vi "RyanChargeDischargeCycling - Copy.vi"() -> ()   [LabVIEW 2020]
uses:
  <instrlib>/NH Research Regenerative Test Series/Public/Configure/Output Safety.ctl
  <vilib>/DAQmx/read.llb/DAQmx Read (Analog 1D DBL NChan 1Samp).vi
  <vilib>/DAQmx/miscellaneous.llb/DAQmx Fill In Error Info.vi
  <instrlib>/NH Research Regenerative Test Series/Public/Data/Read (Ave Current).vi
  <instrlib>/NH Research Regenerative Test Series/Public/Data/Low Level/Fetch (Ave Voltage).vi
  <instrlib>/NH Research Regenerative Test Series/Public/Data/Low Level/Fetch (Ave True Power).vi
  <instrlib>/NH Research Regenerative Test Series/NH Research Regenerative Test Series.lvlib
panel:
  out "Waveform Chart 2":dbl(graph)
  out "Gauge":dbl(knob) scale=0.0..10.0
  out "Boolean":bool
  out "Waveform Chart":dbl(graph)
  in  "Charge Stop":bool
  in  "Post Discharge Wait Time 2":dbl
  out "Discharge Rest Voltage":dbl
  out "Status Byte Register 4":T1
  out "Post Discharge Wait Time Elaspsed":dbl caption="Elapsed Time (s)"
  in  "Discharge Current":dbl
  out "Cycle Index":dbl
  in  "Cycles":dbl
  in  "Discharge Voltage Setpoint":dbl
  out "Task error out":errorcluster
  out "String":string
  out "Filename Out 3":path caption="Filename Out"
  in  "Discharge Data File Name .lvm":path
  out "Ave Current (A) 3":dbl
  out "Ave Voltage (V) 3":dbl
  out "Ave True Power (W) 3":dbl
  out "Status Byte Register 3":T1
  out "Voltage Compare":dbl
  out "Battemp":dbl
  out "AmbientTemp":dbl
  in  "Post Charge Wait Time":dbl
  out "Charge Rest Voltage":dbl
  out "Status Byte Register 2":T1
  out "WaitElapsed Time (s)":dbl caption="Elapsed Time (s)"
  in  "Output Safety":T2
  out "Filename Out":path
  in  "DAQmx Task Name":refnum<k21>
  in  "Charging Data File Name .lvm":path
  in  "Charge Current Cutoff":dbl
  out "Ave Current (A)":dbl
  out "Ave Voltage (V)":dbl
  out "Ave True Power (W)":dbl
  out "Status Byte Register":T1
  out "Battemp":dbl
  out "AmbientTemp":dbl
  in  "Logical Instrument Number":u32=1
  in  "Charge Current":dbl format="%#.6g"
  in  "Charge Voltage":dbl format="%#.6g"
  in  "Battery Detect Voltage (0V)":dbl format="%#.6g"
  in  "VISA resource name":refnum<visa-resource-name>
  # "T couples need calibration"
  # "Dont know which is which"
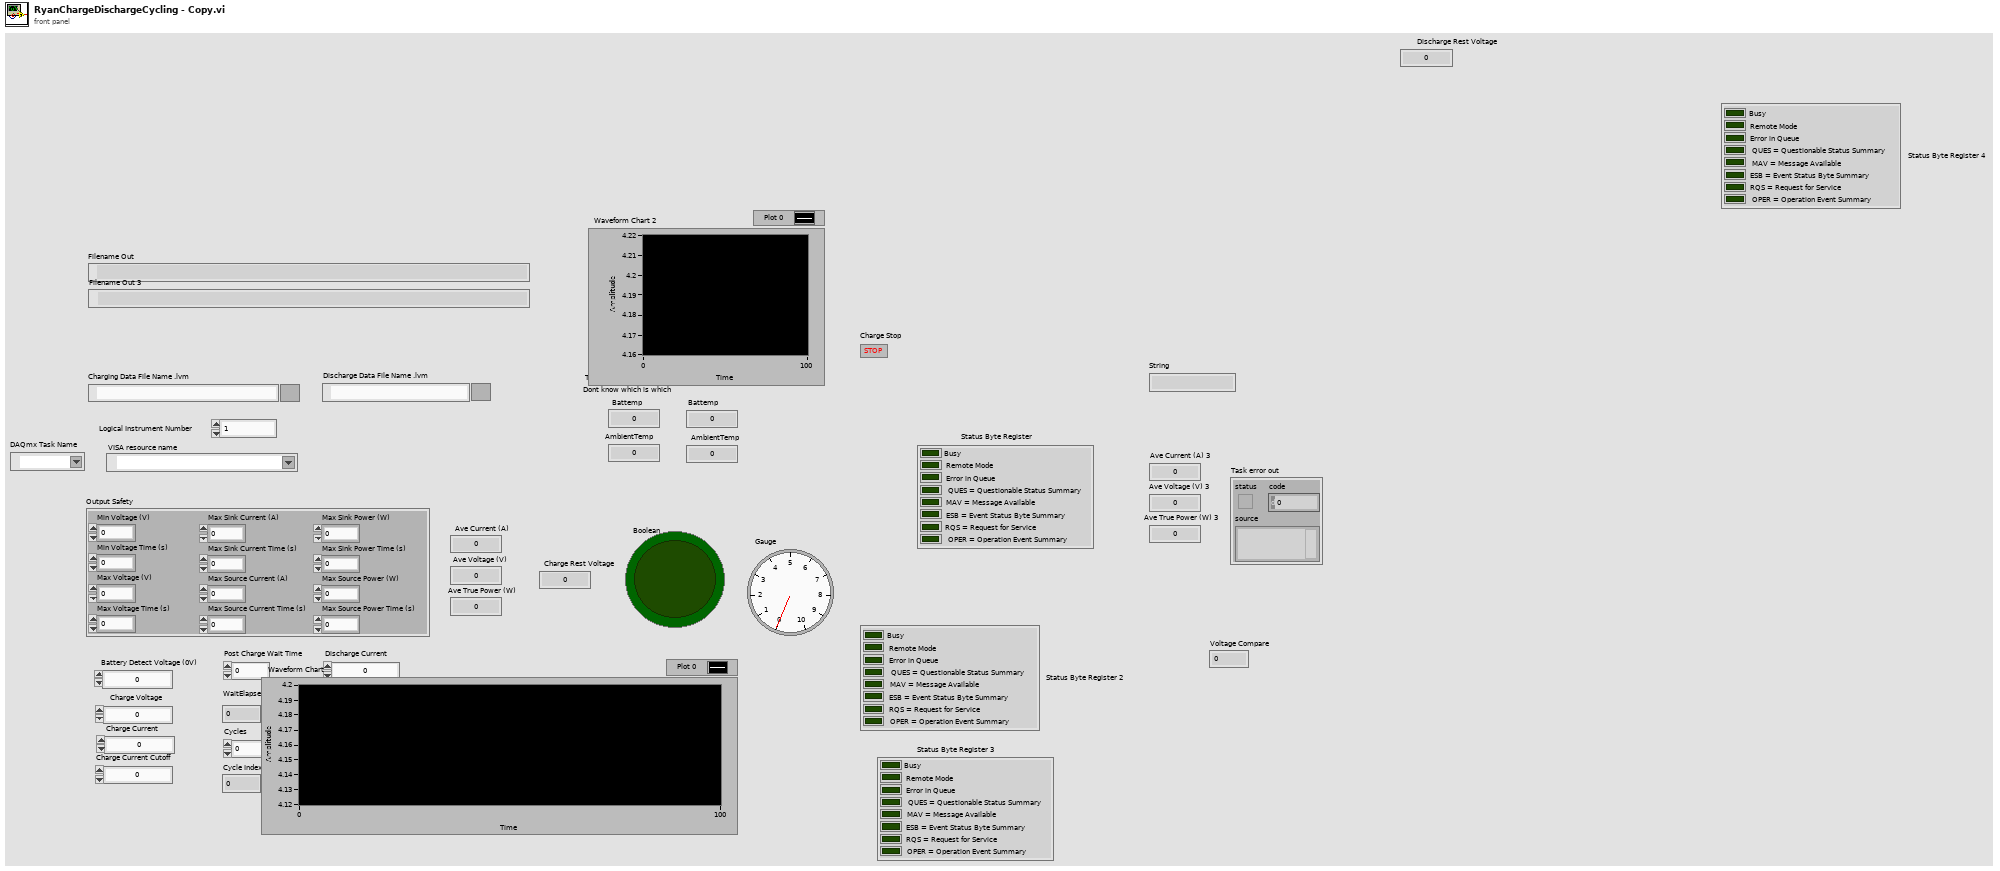
[diagram p1: front panel]
types:
  T1 = cluster{"Busy":bool, "Remote Mode":bool, "Error in Queue":bool, "QUES = Questionable Status Summary":bool, "MAV = Message Available":bool, "ESB = Event Status Byte Summary":bool, "RQS = Request for Service":bool, "OPER = Operation Event Summary":bool}
  T2 = typedef "NH Research Regenerative Test Series.lvlib/Output Safety.ctl" = cluster{"Min Voltage (V)":dbl, "Min Voltage Time (s)":dbl, "Max Voltage (V)":dbl, "Max Voltage Time (s)":dbl, "Max Sink Current (A)":dbl, "Max Sink Current Time (s)":dbl, "Max Source Current (A)":dbl, "Max Source Current Time (s)":dbl, "Max Sink Power (W)":dbl, "Max Sink Power Time (s)":dbl, "Max Source Power (W)":dbl, "Max Source Power Time (s)":dbl}
  T3 = cluster{"data[0]":dbl, "data[1]":dbl, "data[2]":dbl, "data[3]":dbl, "data[4]":dbl, "data[5]":dbl, "data[6]":dbl, "data[7]":dbl, "data[8]":dbl}
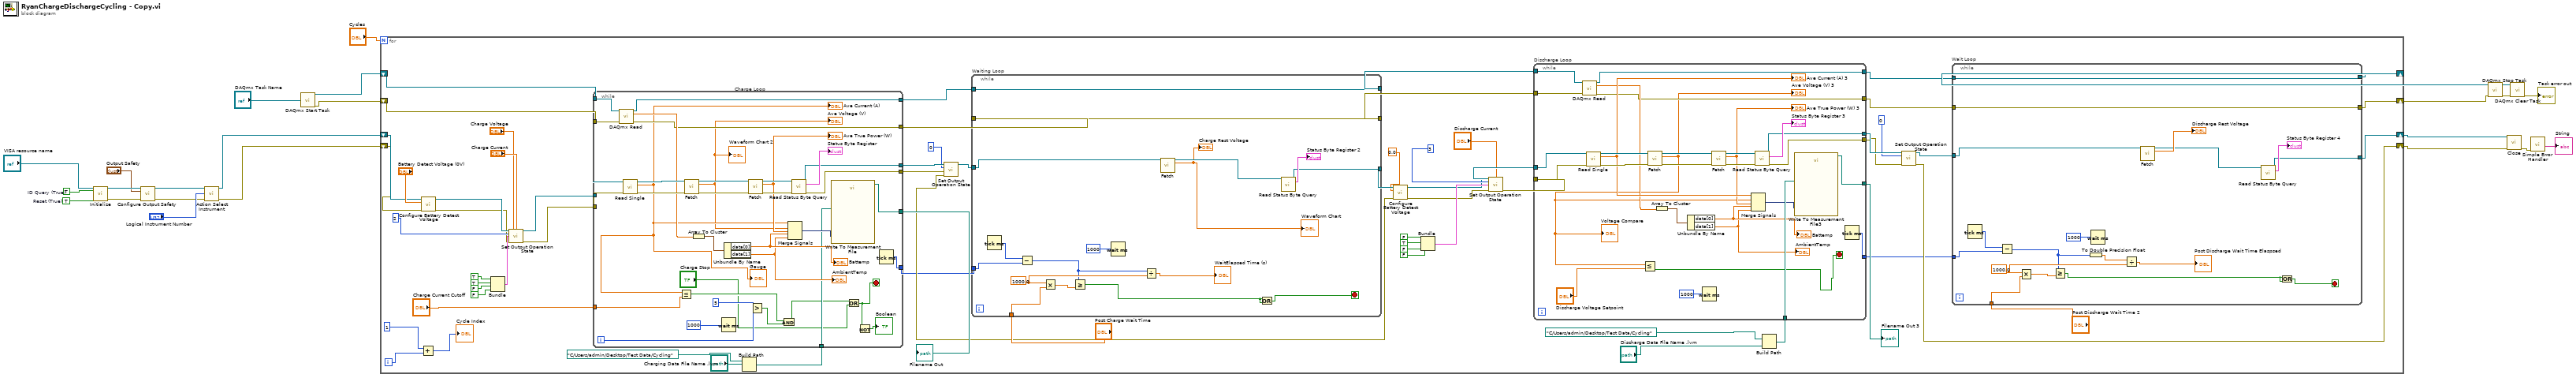
[diagram p0: block diagram]
diagram:
  w23 = TRUE  # ID Query (True)
  w22 = TRUE  # Reset (True)
  n1 = call <vilib>:"Initialize.vi"("VISA resource name"="VISA resource name", "ID Query (True)"=w23, "Reset (True)"=w22) -> ("VISA resource name out"=w21:refnum<visa-resource-name>, "error out"=w20:errorcluster)  [unwired: 11 in]
  n2 = call <vilib>:"Configure Output Safety.vi"("VISA resource name"=w21, "Output Safety"="Output Safety", "error in (no error)"=w20) -> ("VISA resource name out"=w17:refnum<visa-resource-name>, "error out"=w13:errorcluster)  [unwired: 11 in]
  n3 = call <instrlib>:"Action Select Instrument.vi"("VISA resource name"=w17, "Logical Instrument Number"="Logical Instrument Number", "error in (no error)"=w13) -> ("VISA resource name out"=w4:refnum<visa-resource-name>, "error out"=w3:errorcluster)  [unwired: 11 in]
  n4 = call <vilib>:"DAQmx Start Task.vi"("task/channels in"="DAQmx Task Name") -> ("task out"=w15:refnum<k21>, "error out"=w14:errorcluster)  [unwired: 13 in]
  n5 = for {
    N: "Cycles" -> [_]
    shift-right: [w36] -> w2
    shift-left: w4 -> [w48]
    shift-right: [w41] -> w1
    shift-left: w3 -> [w46]
    shift-right: [w34] -> w7
    shift-left: w15 -> [w88]
    shift-right: [w35] -> w6
    shift-left: w14 -> [w87]
    i -> [w43]
    n6 = Add(x=1, y=w43) -> (x+y=→"Cycle Index":i32)
    n7 = call <vilib>:"Configure Battery Detect Voltage.vi"("VISA resource name"=w48, "Battery Detect Voltage (0V)"="Battery Detect Voltage (0V)", "error in (no error)"=w46) -> ("VISA resource name out"=w47:refnum<visa-resource-name>, "error out"=w45:errorcluster)  [unwired: 11 in]
    n8 = Bundle(TRUE, TRUE, FALSE, FALSE) -> (w49:cluster{bool, bool, bool, bool})  [unwired: 1 in]
    n9 = call <vilib>:"Set Output Operation State.vi"("VISA resource name"=w47, "Voltage Setpoint (0 V)"="Charge Voltage", "Current Setpoint (0 A)"="Charge Current", "Mode (0: Off)"=2, "Enable"=w49, "error in (no error)"=w45) -> ("VISA resource name out"=w58:refnum<visa-resource-name>, "error out"=w57:errorcluster)  [unwired: 8 in]
    n10 = Build Path(base path=path "C:/Users/admin/Desktop/Test Data/Cycling", name or relative path="Charging Data File Name .lvm") -> (appended path=w28:path)
    n11 = while "Charge Loop" {
      tunnel: w58 -> [w183]
      tunnel: w57 -> [w182]
      tunnel: [w180] -> w65
      tunnel: [w179] -> w64
      tunnel: "Charge Current Cutoff" -> [w169]
      tunnel: w28 -> [w160]
      tunnel: w88 -> [w177]
      tunnel: [w173] -> w84
      tunnel: [w172] -> w83
      tunnel: w87 -> [w171]
      tunnel: [w170] -> w89
      tunnel: [w161] -> w32
      i -> [w162]
      stop <- w156 stop-if-true
      n12 = call-poly <vilib>:"DAQmx Read.vi"("task/channels in"=w177, "error in"=w171) -> ("task out"=w173:refnum<k21>, "data"=w176:dbl[], "error out"=w172:errorcluster)  [unwired: 11 in]
      n13 = call-poly <instrlib>:"Read Single.vi"("VISA resource name"=w183, "error in (no error)"=w182) -> ("VISA resource name out"=w188:refnum<visa-resource-name>, "Ave Current (A)"=w155:dbl, "error out"=w189:errorcluster)  [unwired: 11 in]
      "Ave Current (A)" <- w155
      "Gauge" <- w155
      n14 = Less Or Equal?(x=w155, y=w169) -> (x <= y?=w164:bool)
      n15 = call-poly <instrlib>:"Fetch.vi"("VISA resource name"=w188, "error in (no error)"=w189) -> ("VISA resource name out"=w187:refnum<visa-resource-name>, "Ave Voltage (V)"=w154:dbl, "error out"=w186:errorcluster)  [unwired: 11 in]
      "Ave Voltage (V)" <- w154
      "Waveform Chart 2" <- w154
      n16 = Array To Cluster(array=w176) -> (cluster=w175:T3)
      n17 = Wait (ms)(milliseconds to wait=1000) -> ()  [unwired: 1 out]
      n18 = Unbundle By Name(w175) -> ("data[0]"=w168:dbl, "data[1]"=w167:dbl)
      "Battemp" <- w168
      "AmbientTemp" <- w167
      n19 = call-poly <instrlib>:"Fetch.vi"("VISA resource name"=w187, "error in (no error)"=w186) -> ("VISA resource name out"=w185:refnum<visa-resource-name>, "Ave True Power (W)"=w178:dbl, "error out"=w184:errorcluster)  [unwired: 11 in]
      "Ave True Power (W)" <- w178
      n20 = Greater?(x=w162, y=5) -> (0:w163:bool)
      n21 = And(x=w164, y=w163) -> (x .and. y?=w159:bool)
      n22 = Merge Signals "Merge Signals"(w155, w154, w178, w168, w167) -> (w174:dynamicdata)
      n23 = call <instrlib>:"Read Status Byte Query.vi"("VISA resource name"=w185, "error in (no error)"=w184) -> ("VISA resource name out"=w180:refnum<visa-resource-name>, "Status Byte Register"=→"Status Byte Register":T1, "error out"=w179:errorcluster)  [unwired: 11 in]
      n24 = call "Write To Measurement File"("Signals"=w174, "Filename"=w160) -> ("Filename Out"=w170:path)  [unwired: 15 in, 2 out]
      n25 = Or(x=w159, y="Charge Stop") -> (x .or. y?=w156:bool)
      n26 = Not(x=w156) -> (.not. x?=→"Boolean":bool)
      n27 = Tick Count (ms)() -> (millisecond timer value=w161:u32)
    }
    "Filename Out" <- w89
    n28 = call <vilib>:"Set Output Operation State.vi"("VISA resource name"=w65, "Mode (0: Off)"=0, "error in (no error)"=w64) -> ("VISA resource name out"=w61:refnum<visa-resource-name>, "error out"=w63:errorcluster)  [unwired: 11 in]
    n29 = while "Waiting Loop" {
      tunnel: [w152] -> w68
      tunnel: "Post Charge Wait Time" -> [w151]
      tunnel: w32 -> [w147]
      tunnel: [w142] -> w79
      tunnel: [w143] -> w80
      tunnel: w83 -> [w142]
      tunnel: w84 -> [w143]
      tunnel: w61 -> [w141]
      stop <- w139 stop-if-true
      w148 = 1000.0
      n30 = Tick Count (ms)() -> (millisecond timer value=w146:u32)
      n31 = Subtract(x=w146, y=w147) -> (x-y=w145:u32)
      n32 = Multiply(x=w148, y=w151) -> (x*y=w150:dbl)
      n33 = Greater Or Equal?(x=w145, y=w150) -> (x >= y?=w138:bool)
      n34 = Wait (ms)(milliseconds to wait=1000) -> ()  [unwired: 1 out]
      n35 = Divide(x=w145, y=w148) -> (x/y=→"WaitElapsed Time (s)":dbl)
      n36 = call-poly <instrlib>:"Fetch.vi"("VISA resource name"=w141) -> ("VISA resource name out"=w140:refnum<visa-resource-name>, "Ave Voltage (V)"=→"Charge Rest Voltage" →"Waveform Chart":dbl)  [unwired: 12 in, 1 out]
      n37 = Or(x=w138, y=w138) -> (x .or. y?=w139:bool)
      n38 = call <instrlib>:"Read Status Byte Query.vi"("VISA resource name"=w140) -> ("VISA resource name out"=w152:refnum<visa-resource-name>, "Status Byte Register"=→"Status Byte Register 2":T1)  [unwired: 12 in, 1 out]
    }
    n39 = call <vilib>:"Configure Battery Detect Voltage.vi"("VISA resource name"=w68, "Battery Detect Voltage (0V)"=0.0, "error in (no error)"=w63) -> ("VISA resource name out"=w67:refnum<visa-resource-name>, "error out"=w69:errorcluster)  [unwired: 11 in]
    n40 = Bundle(FALSE, TRUE, FALSE, FALSE) -> (w74:cluster{bool, bool, bool, bool})  [unwired: 1 in]
    n41 = call <vilib>:"Set Output Operation State.vi"("VISA resource name"=w67, "Current Setpoint (0 A)"="Discharge Current", "Mode (0: Off)"=3, "Enable"=w74, "error in (no error)"=w69) -> ("VISA resource name out"=w81:refnum<visa-resource-name>, "error out"=w82:errorcluster)  [unwired: 9 in]
    n42 = Build Path(base path=path "C:/Users/admin/Desktop/Test Data/Cycling", name or relative path="Discharge Data File Name .lvm") -> (appended path=w26:path)
    n43 = while "Discharge Loop" {
      tunnel: w81 -> [w130]
      tunnel: w82 -> [w129]
      tunnel: [w127] -> w72
      tunnel: [w126] -> w71
      tunnel: w26 -> [w123]
      tunnel: w80 -> [w122]
      tunnel: [w118] -> w39
      tunnel: [w117] -> w38
      tunnel: w79 -> [w116]
      tunnel: [w115] -> w40
      tunnel: [w110] -> w31
      stop <- w108 stop-if-true
      n44 = call-poly <vilib>:"DAQmx Read.vi"("task/channels in"=w122, "error in"=w116) -> ("task out"=w118:refnum<k21>, "data"=w121:dbl[], "error out"=w117:errorcluster)  [unwired: 11 in]
      n45 = call-poly <instrlib>:"Read Single.vi"("VISA resource name"=w130, "error in (no error)"=w129) -> ("VISA resource name out"=w135:refnum<visa-resource-name>, "Ave Current (A)"=w125:dbl, "error out"=w136:errorcluster)  [unwired: 11 in]
      "Ave Current (A) 3" <- w125
      n46 = call-poly <instrlib>:"Fetch.vi"("VISA resource name"=w135, "error in (no error)"=w136) -> ("VISA resource name out"=w134:refnum<visa-resource-name>, "Ave Voltage (V)"=w114:dbl, "error out"=w133:errorcluster)  [unwired: 11 in]
      "Ave Voltage (V) 3" <- w114
      "Voltage Compare" <- w114
      n47 = Less Or Equal?(x=w114, y="Discharge Voltage Setpoint") -> (x <= y?=w108:bool)
      n48 = Array To Cluster(array=w121) -> (cluster=w120:T3)
      n49 = Unbundle By Name(w120) -> ("data[0]"=w113:dbl, "data[1]"=w112:dbl)
      "Battemp" <- w113
      "AmbientTemp" <- w112
      n50 = Wait (ms)(milliseconds to wait=1000) -> ()  [unwired: 1 out]
      n51 = call-poly <instrlib>:"Fetch.vi"("VISA resource name"=w134, "error in (no error)"=w133) -> ("VISA resource name out"=w132:refnum<visa-resource-name>, "Ave True Power (W)"=w124:dbl, "error out"=w131:errorcluster)  [unwired: 11 in]
      "Ave True Power (W) 3" <- w124
      n52 = Merge Signals "Merge Signals"(w125, w114, w124, w113, w112) -> (w119:dynamicdata)
      n53 = call <instrlib>:"Read Status Byte Query.vi"("VISA resource name"=w132, "error in (no error)"=w131) -> ("VISA resource name out"=w127:refnum<visa-resource-name>, "Status Byte Register"=→"Status Byte Register 3":T1, "error out"=w126:errorcluster)  [unwired: 11 in]
      n54 = call "Write To Measurement File3"("Signals"=w119, "Filename"=w123) -> ("Filename Out"=w115:path)  [unwired: 15 in, 2 out]
      n55 = Tick Count (ms)() -> (millisecond timer value=w110:u32)
    }
    "Filename Out 3" <- w40
    n56 = call <vilib>:"Set Output Operation State.vi"("VISA resource name"=w72, "Mode (0: Off)"=0, "error in (no error)"=w71) -> ("VISA resource name out"=w37:refnum<visa-resource-name>, "error out"=w41:errorcluster)  [unwired: 11 in]
    n57 = while "Wait Loop" {
      tunnel: [w106] -> w36
      tunnel: "Post Discharge Wait Time 2" -> [w104]
      tunnel: w31 -> [w100]
      tunnel: [w97] -> w35
      tunnel: [w98] -> w34
      tunnel: w38 -> [w97]
      tunnel: w39 -> [w98]
      tunnel: w37 -> [w96]
      stop <- w91 stop-if-true
      w101 = 1000.0
      n58 = Tick Count (ms)() -> (millisecond timer value=w99:u32)
      n59 = Subtract(x=w99, y=w100) -> (x-y=w94:u32)
      n60 = Multiply(x=w101, y=w104) -> (x*y=w103:dbl)
      n61 = Greater Or Equal?(x=w94, y=w103) -> (x >= y?=w90:bool)
      n62 = To Double Precision Float(number=w94) -> (double precision float=w93:dbl)
      n63 = Wait (ms)(milliseconds to wait=u32 1000) -> ()  [unwired: 1 out]
      n64 = Divide(x=w93, y=w101) -> (x/y=→"Post Discharge Wait Time Elaspsed":dbl)
      n65 = call-poly <instrlib>:"Fetch.vi"("VISA resource name"=w96) -> ("VISA resource name out"=w95:refnum<visa-resource-name>, "Ave Voltage (V)"=→"Discharge Rest Voltage":dbl)  [unwired: 12 in, 1 out]
      n66 = call <instrlib>:"Read Status Byte Query.vi"("VISA resource name"=w95) -> ("VISA resource name out"=w106:refnum<visa-resource-name>, "Status Byte Register"=→"Status Byte Register 4":T1)  [unwired: 12 in, 1 out]
      n67 = Or(x=w90, y=w90) -> (x .or. y?=w91:bool)
    }
  }
  n68 = call <vilib>:"DAQmx Stop Task.vi"("task/channels in"=w7, "error in"=w6) -> ("task out"=w11:refnum<k21>, "error out"=w10:errorcluster)  [unwired: 12 in]
  n69 = call <instrlib>:"Close.vi"("VISA resource name"=w2, "error in (no error)"=w1) -> ("error out"=w8:errorcluster)  [unwired: 13 in]
  n70 = call <vilib>:"DAQmx Clear Task.vi"("task in"=w11, "error in"=w10) -> ("error out"=→"Task error out":errorcluster)  [unwired: 13 in]
  n71 = call <vilib>:"Simple Error Handler.vi"("error in (no error)"=w8) -> ("source out"=→"String":string)  [unwired: 4 in, 4 out]
